vi "Close Device.vi"(0 "session in":refnum<class "Digitizer Control.lvclass">, 5 "error in (no error)":errorcluster) -> (19 "error out":errorcluster)   [LabVIEW 2021, in "Digitizer Control.lvclass"]
doc: "Closes the FlexRIO Transceiver opened by the <B>Open Device.vi</B>.\n\nThis VI runs normally even if an error code is passed on the <B>error in</B> input.\n\nInput:\n\n<B>session in</B>: The device session created by the <B>Open Device.vi</B>."
uses:
  Digitizer Control.lvclass
  Digitizer Control.lvclass/Digitizer Control.ctl
  <vilib>/FPGAPlugInAG/Dynamic/niLvFpga_Close_Dynamic.vi
  <vilib>/rvi/interface/nirviCloseFPGA/nirviCloseFPGA.xnode
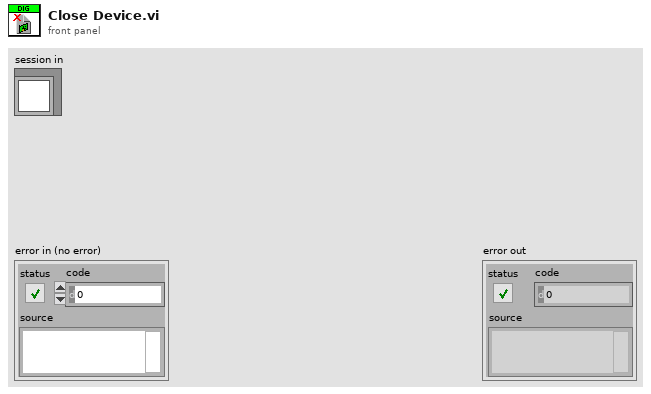
[diagram p1: front panel]
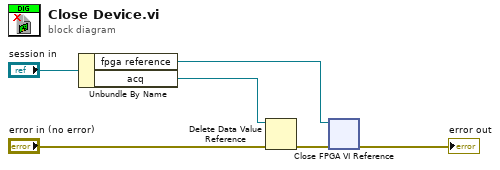
[diagram p0: block diagram]
diagram:
  n1 = Unbundle By Name("session in") -> ("fpga reference"=w2:refnum<k20>, "acq"=w3:refnum<data-value>)
  n2 = Delete Data Value Reference(data value reference=w3, error in="error in (no error)") -> (error out=w6:errorcluster)  [unwired: 1 out]
  n3 = xnode "Close FPGA VI Reference"("FPGA VI Reference In"=w2, "error in"=w6) -> ("error out"=→"error out":errorcluster)
